vi "Bind STR parameter.vi"(4 "error in (no error)":errorcluster, 5 "Database String Length (255)":i32=255, 6 "Parameter":string, 7 "Statement Refnum":T1) -> (0 "error out":errorcluster, 3 "Statement Refnum":T1)   [LabVIEW 2011]
doc: "Charge le paramètre de type string dans la pile et l'interpète comme champ texte (limité à 255 caractères)"
uses:
  SQL Controls/Statement Refnum.ctl
  Odbc32.dll
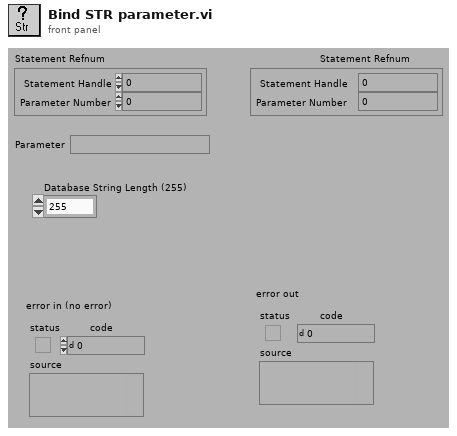
[diagram p1: front panel]
types:
  T1 = typedef "Statement Refnum.ctl" = cluster{"Statement Handle":i32, "Parameter Number":u16}
  T2 = enum16{"NOPE", "SQL_HANDLE_ENV", "SQL_HANDLE_DBC", "SQL_HANDLE_STMT", "SQL_HANDLE_DESC"}
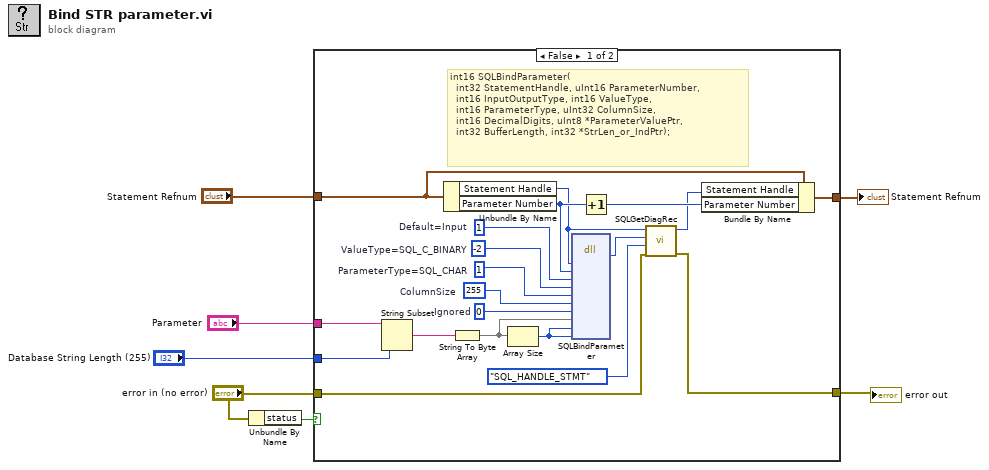
[diagram p0: block diagram]
diagram:
  n1 = Unbundle By Name("error in (no error)") -> ("status"=w2:bool)
  n2 = case shown="False" w2 {
    tunnel: "Statement Refnum" -> [w27 w29]
    tunnel: [w23 w29] -> w6
    tunnel: "Parameter" -> [w10 _]
    tunnel: "error in (no error)" -> [w13 w28]
    tunnel: [w12 w28] -> w4
    tunnel: "Database String Length (255)" -> [w8 _]
    frame False {
      w19 = i16 1  # ParameterType=SQL_CHAR
      w21 = u32 255  # ColumnSize
      w22 = i16 0  # Ignored
      w20 = i16 -2  # ValueType=SQL_C_BINARY
      w25 = i16 1  # Default=Input
      # "int16 SQLBindParameter(\n  int32 StatementHandle, uInt16 ParameterNumber, \n  int16 InputOutputType, int16 ValueType, \n  int16 ParameterType, uInt32 ColumnSize, \n  int16 DecimalDigits, uInt8 *ParameterValuePtr, \n  int32 BufferLength, int32 *StrLen_or_IndPtr);"
      n3 = String Subset(string=w10, length (rest)=w8) -> (substring=w9:string)  [unwired: 1 out]
      n4 = Unbundle By Name(w27) -> ("Statement Handle"=w15:i32, "Parameter Number"=w26:u16)
      n5 = String To Byte Array(string=w9) -> (unsigned byte array=w18:u8[])
      n6 = Array Size(array=w18) -> (size(s)=w17:i32)
      n7 = dll-call lib="Odbc32.dll" fn="SQLBindParameter"("StatementHandle"=w15, "ParameterNumber"=w26, "InputOutputType"=w25, "ValueType"=w20, "ParameterType"=w19, "ColumnSize"=w21, "DecimalDigits"=w22, "ParameterValuePtr"=w18, "BufferLength"=w17, "StrLen_or_IndPtr"=w17) -> (w16:i16)  [unwired: 11 in, 4 out]
      n8 = Increment(x=w26) -> (x+1=w24:u16)
      n9 = call "SQLGetDiagRec.vi"("error in (no error)"=w13, "HandleType"=T2."SQL_HANDLE_STMT", "Status (SQL_SUCCESS=0)"=w16, "Input Handle"=w15) -> ("error out"=w12:errorcluster, "Output Handle"=w14:i32)  [unwired: 2 out]
      n10 = Bundle By Name(cluster=w27, "Statement Handle"=w14, "Parameter Number"=w24) -> (w23:T1)
    }
    frame True {
    }
  }
  "Statement Refnum" <- w6
  "error out" <- w4
